vi "HW_6p1_Task3_PRADHASK.vi"() -> ()   [LabVIEW 2016]
panel:
  out "Category":string
  in  "Haemoglobin A1c (%)":dbl
  in  "Fasting blood glucose (mg/dL)":dbl
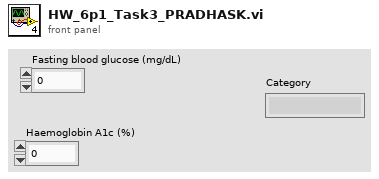
[diagram p1: front panel]
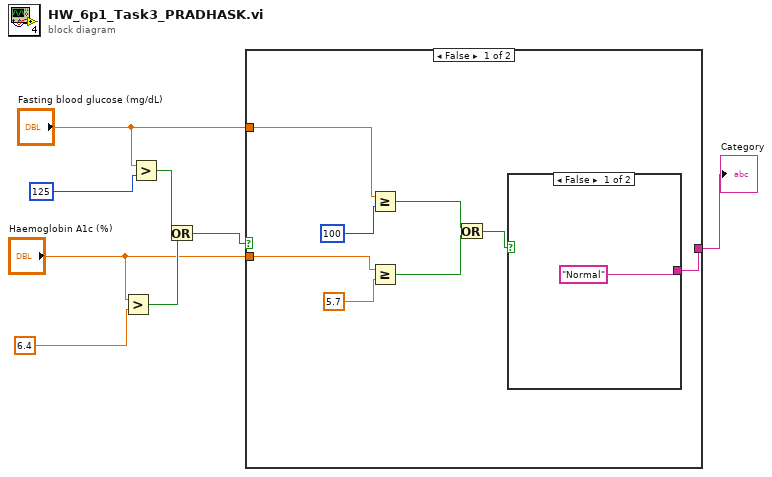
[diagram p0: block diagram]
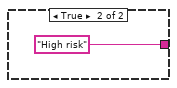
[diagram p2: hidden frame]
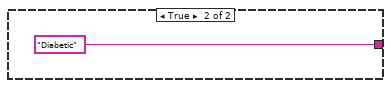
[diagram p3: hidden frame]
diagram:
  n1 = Greater?(x="Haemoglobin A1c (%)", y=6.4) -> (0:w5:bool)
  n2 = Greater?(x="Fasting blood glucose (mg/dL)", y=125) -> (0:w6:bool)
  n3 = Or(x=w6, y=w5) -> (x .or. y?=w4:bool)
  n4 = case shown="False" w4 {
    tunnel: [w9 "Diabetic"] -> w3
    tunnel: "Fasting blood glucose (mg/dL)" -> [w16 _]
    tunnel: "Haemoglobin A1c (%)" -> [w14 _]
    frame False {
      n5 = Greater Or Equal?(x=w16, y=100) -> (x >= y?=w11:bool)
      n6 = Greater Or Equal?(x=w14, y=5.7) -> (x >= y?=w12:bool)
      n7 = Or(x=w11, y=w12) -> (x .or. y?=w10:bool)
      n8 = case shown="False" w10 {
        tunnel: ["Normal" "High risk"] -> w9
        frame False {
        }
        frame True {
        }
      }
    }
    frame True {
    }
  }
  "Category" <- w3
